vi "Stop Core.vi"(10 "final error code":i32, 11 "Network Actor in":refnum<class "Client LNA.lvclass">) -> (3 "Network Actor out":refnum<class "Client LNA.lvclass">)   [LabVIEW 2026, in "Client LNA.lvlib" / "Client LNA.lvclass"]
doc: "Defines what the actor does before it stops. Use the <B>final error code</B> input to determine whether the actor shut down normally. By default, a value of 43 indicates the actor stopped normally. Any other value indicates the actor stopped due to an error. However, descendants of Actor.lvclass can override Actor.lvclass:Handle Error.vi to change this behavior.\n\nBy default, this method does nothing. A descendant class may override it to define behavior, such as shutting down any processes the actor initiated in its override of Actor.lvclass:Actor Core.vi."
uses:
  Client LNA.lvclass
  Client LNA.lvclass/Client LNA.ctl
  C:/Users/E2013170/Documents/GitHub/Measurement-Utility-Reference/recovery/packages/ni_lib_linked_network_actor-1.2.0.19-9492AF5A82/File Group 0/vi.lib/NI/Actors/Linked Network Actor/Linked Network Actor/Linked Network Actor.lvclass
  C:/Program Files/National Instruments/LabVIEW 2026/vi.lib/ActorFramework/Actor/Actor.lvclass
  C:/Users/E2013170/Documents/GitHub/Measurement-Utility-Reference/components/HAL-MAL-Application/Source/Framework/Client/Client LNA/Client LNA.lvclass
  recovery/packages/ni_lib_linked_network_actor-1.2.0.19-9492AF5A82/File Group 0/vi.lib/NI/Actors/Linked Network Actor/Linked Network Actor/Linked Network Actor.lvclass
  <vilib>/ActorFramework/Actor/Actor.lvclass
  Client Controller/Messages/LNA Stopped Msg/LNA Stopped Msg.lvclass
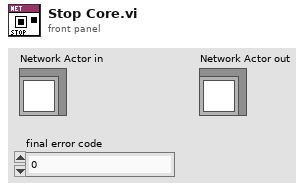
[diagram p1: front panel]
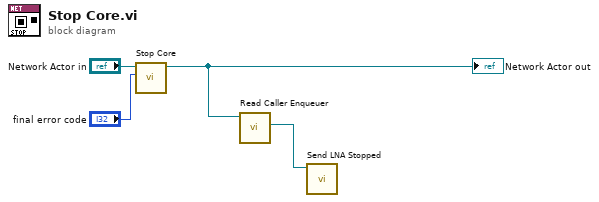
[diagram p0: block diagram]
diagram:
  n1 = call-parent "Stop Core.vi"("final error code"="final error code", "Network Actor in"="Network Actor in") -> ("Network Actor out"=w1:refnum<class "Client LNA.lvclass">)  [unwired: 9 in]
  "Network Actor out" <- w1
  n2 = call <vilib>:"Read Caller Enqueuer.vi"("Actor"=w1) -> ("Caller Enqueuer"=w2:refnum<class "Message Enqueuer.lvclass">)  [unwired: 10 in]
  n3 = call "Send LNA Stopped.vi"("Message Enqueuer"=w2) -> ()  [unwired: 9 in, 2 out]
